vi "Destruct.vi"(8 "Error in (no error)":errorcluster, 11 "Log in":refnum<class "Log.lvclass">) -> (0 "Error out":errorcluster)   [LabVIEW 2011, in "Log.lvclass"]
uses:
  Log.lvclass
  Log.lvclass/Log.ctl
  Writer/LogWriterInterface/LogWriterInterface.lvclass
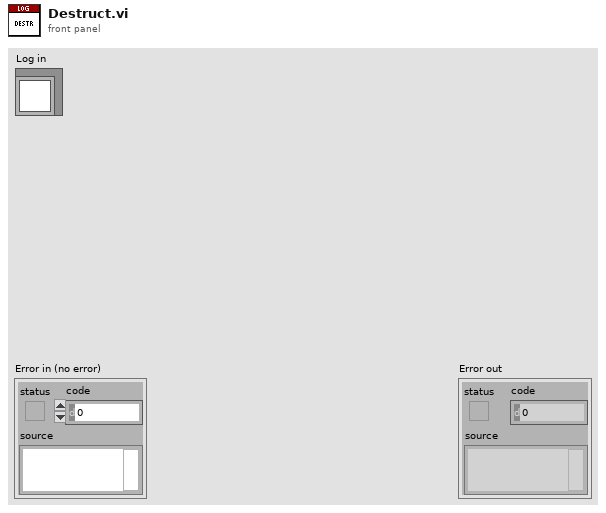
[diagram p1: front panel]
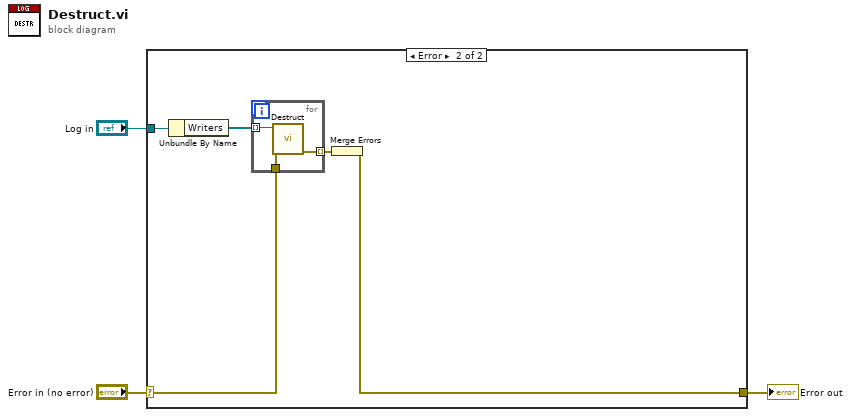
[diagram p0: block diagram]
diagram:
  n1 = case shown="Error" "Error in (no error)" {
    selector: "Error in (no error)" -> [w4 w6]
    tunnel: [w4 w5] -> w2
    tunnel: "Log in" -> [_ w9]
    frame No Error {
    }
    frame Error {
      n2 = Unbundle By Name(w9) -> ("Writers"=w8:refnum<class "LogWriterInterface.lvclass">[])
      n3 = for {
        tunnel: w8 -> [w12] mode=indexing
        tunnel: w6 -> [w11]
        tunnel: [w10] -> w7 mode=indexing
        n4 = call-dynamic "Destruct.vi"("Error in (no error)"=w11, "LogWriterInterface in"=w12) -> ("Error out"=w10:errorcluster)  [unwired: 8 in, 1 out]
      }
      n5 = Merge Errors(w7) -> (w5:errorcluster)
    }
  }
  "Error out" <- w2
